vi "CoordinatorTrigger.vi"(8 "error in (no error)":errorcluster) -> (0 "error out":errorcluster)   [LabVIEW 2013, in "AnimatorXControl.xctl"]
uses:
  AnimatorXControl.xctl
  AnimatorCoordinator.vi
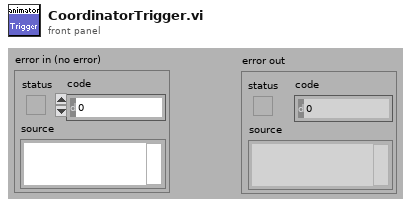
[diagram p1: front panel]
types:
  T1 = enum32{"Bad", "Idle", "Run top level", "Running"}
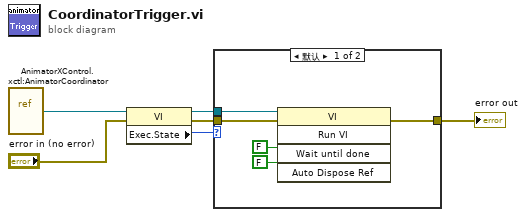
[diagram p0: block diagram]
diagram:
  n1 = vi-ref "AnimatorXControl.xctl:AnimatorCoordinator.vi"() -> (w6:refnum<vi>)
  n2 = property class="VI"(reference=w6, error in="error in (no error)") -> (reference out=w4:refnum<vi>, error out=w3:errorcluster, "Exec.State"=w5:T1)
  n3 = case shown="默认" w5 {
    tunnel: w4 -> [w11 _]
    tunnel: w3 -> [w8 w12]
    tunnel: [w7 w12] -> w1
    frame Default {
      n4 = invoke class="VI" method="Run VI"(reference=w11, error in=w8, "Wait until done"=FALSE ("Wait Until Done"), "Auto Dispose Ref"=FALSE ("Auto Dispose Reference")) -> (error out=w7:errorcluster)  [unwired: 1 in, 4 out]
    }
    frame "Run top level", "Running" {
    }
  }
  "error out" <- w1
